vi "RangeBuffer.vi"(4 "DATA Input":dbl[][](array[numeric]), 5 "WindowSize":i32, 6 "Fetch Rate":i32) -> (0 "Raw Data":dbl[](array[numeric]), 1 "Mean Average":dbl[](array[numeric]), 2 "Standard Deviation":dbl[](array[numeric]))   [LabVIEW 2012]
uses:
  <vilib>/Analysis/baseanly.llb/Mean (DBL).vi
  <vilib>/Analysis/NI_AALBase.lvlib
panel:
  # "This VI calculates an approximate of the standard deviation and \nthe mean of the signal over a predefined window.\n\nThe rotating buffer only stores the min and max during each \nfetch and it is assumed that the standard deviation of the min-max\nsignals are equal to the standard deviation of the real signal."
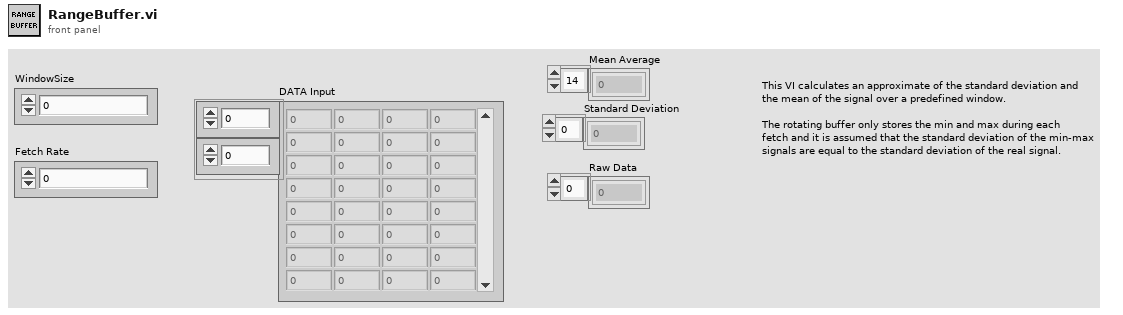
[diagram p1: front panel]
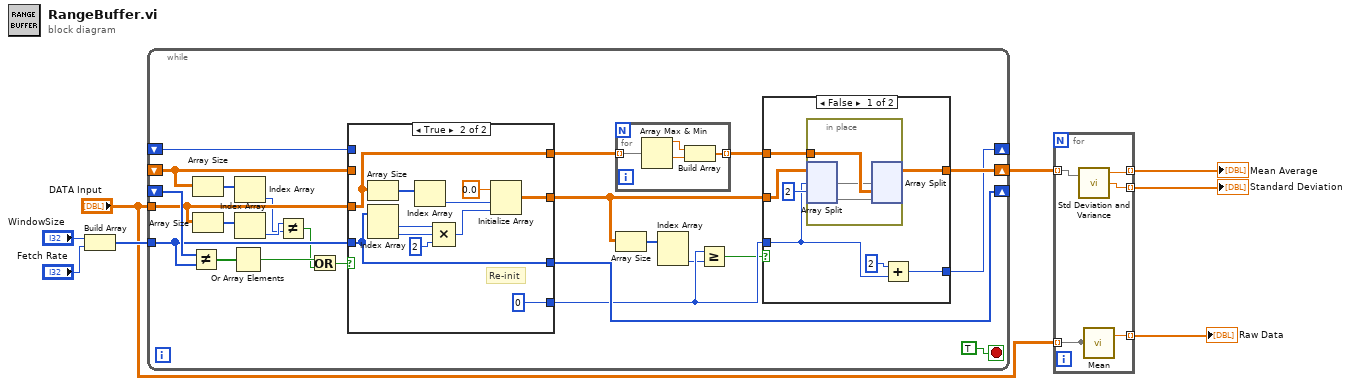
[diagram p0: block diagram]
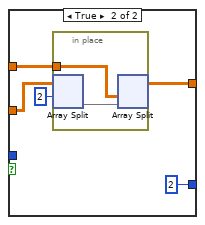
[diagram p2: hidden frame]
diagram:
  n1 = Build Array("WindowSize", "Fetch Rate") -> (w6:i32[])
  n2 = while {
    tunnel: w6 -> [w28]
    shift-right: [w27] -> _
    shift-left: _ -> [w31]
    shift-right: [w25] -> w3
    shift-left: _ -> [w15]
    tunnel: "DATA Input" -> [w18]
    shift-right: [w19] -> _
    shift-left: _ -> [w26]
    stop <- TRUE stop-if-true
    n3 = Not Equal?(x=w31, y=w28) -> (x != y?=w30:bool[])
    n4 = Array Size(array=w15) -> (size(s)=w16:i32[])
    n5 = Array Size(array=w18) -> (size(s)=w17:i32[])
    n6 = Or Array Elements(Boolean array=w30) -> (logical OR=w29:bool)
    n7 = Index Array(array=w16) -> (element=w13:i32)  [unwired: 1 in]
    n8 = Index Array(array=w17) -> (element=w14:i32)  [unwired: 1 in]
    n9 = Not Equal?(x=w14, y=w13) -> (x != y?=w11:bool)
    n10 = Or(x=w29, y=w11) -> (x .or. y?=w12:bool)
    n11 = case shown="True" w12 {
      tunnel: [w57 w67] -> w27
      tunnel: w28 -> [w57 w67]
      tunnel: w18 -> [w56 w59]
      tunnel: [w54 w60] -> w24
      tunnel: [w56 w59] -> w10
      tunnel: w26 -> [w55 _]
      tunnel: w15 -> [w54 _]
      tunnel: [w55 0] -> w22
      frame False {
      }
      frame True {
        # "Re-init"
        n12 = Array Size(array=w59) -> (size(s)=w62:i32[])
        n13 = Index Array(array=w67) -> (element #1=w66:i32, element #2=w65:i32)  [unwired: 2 in]
        n14 = Index Array(array=w62) -> (element=w61:i32)  [unwired: 1 in]
        n15 = Compound Arithmetic op=MULTIPLY(w66, w65, 2 ("value")) -> (w63:i32)
        n16 = Initialize Array(0.0 ("element"), w61, w63) -> (w60:dbl[][])
      }
    }
    n17 = for {
      tunnel: w10 -> [w53] mode=indexing
      tunnel: [w50] -> w9 mode=indexing
      n18 = Array Max & Min(array=w53) -> (max value=w52:dbl, min value=w51:dbl)  [unwired: 2 out]
      n19 = Build Array(w52, w51) -> (w50:dbl[])
    }
    n20 = Array Size(array=w24) -> (size(s)=w23:i32[])
    n21 = Index Array(array=w23) -> (element #2=w21:i32)  [unwired: 2 in, 1 out]
    n22 = Greater Or Equal?(x=w22, y=w21) -> (x >= y?=w20:bool)
    n23 = case shown="False" w20 {
      tunnel: w9 -> [w38 w47]
      tunnel: [w37 w46] -> w25
      tunnel: w24 -> [w36 w45]
      tunnel: w22 -> [w35 _]
      tunnel: [w34 2] -> w19
      frame False {
        n24 = in-place {
          in-place-border: w38 -> [w41]
          n25 = in-place-split #1(w36, w35, 2) -> (w40:dbl[][], w42:dbl[][])  [unwired: 1 out]
          n26 = in-place-split #1(w40, w41, w42) -> (w37:dbl[][])  [unwired: 2 out]
        }
        n27 = Add(x=2, y=w35) -> (x+y=w34:i32)
      }
      frame True {
        n28 = in-place {
          in-place-border: w47 -> [w48]
          n29 = in-place-split #2(w45, 2) -> (w49:dbl[][])  [unwired: 1 out]
          n30 = in-place-split #2(w48, w49) -> (w46:dbl[][])  [unwired: 1 out]
        }
      }
    }
  }
  n31 = for {
    tunnel: w3 -> [w71] mode=indexing
    tunnel: [w70] -> w4 mode=indexing
    tunnel: [w69] -> w5 mode=indexing
    tunnel: [w73] -> _ mode=indexing
    tunnel: "DATA Input" -> [w73] mode=indexing
    tunnel: [w72] -> w1 mode=indexing
    n32 = call <vilib>:"Std Deviation and Variance.vi"("X"=w71) -> ("mean"=w70:dbl, "standard deviation"=w69:dbl)  [unwired: 1 in, 1 out]
    n33 = call-poly <vilib>:"Mean.vi"("X"=w73) -> ("mean"=w72:dbl)  [unwired: 1 out]
  }
  "Standard Deviation" <- w5
  "Mean Average" <- w4
  "Raw Data" <- w1
